vi "Create Section.vi"(8 "error in":errorcluster, 11 "Node In":refnum<k20>) -> (0 "error out":errorcluster, 2 "Section out":refnum<class "Section.lvclass">, 3 "Node out":refnum<k20>)   [LabVIEW 2024, in "Parser.lvlib" / "Section.lvclass"]
uses:
  Section.lvclass
  C:/Users/kperiyas/Downloads/Parser/Parser/Item/Item.lvclass
  Section.lvclass/Section.ctl
  Item/Item.lvclass/Item.ctl
  Item/Write Child Items.vi
  Item/Write Properties.vi
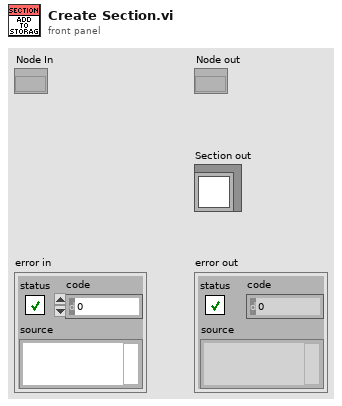
[diagram p1: front panel]
types:
  T1 = cluster{"Errors":cluster{"Key":string, "IsError":bool, "Code":u32, "Message":string}[], "Description":string}
  T2 = typedef "Parser.lvlib/Item.lvclass/Item Type.ctl" = enum16{"Channel", "Section"}
  T3 = cluster{"Name":string, "TypeGUID":string, "Identifier":string}
  T4 = cluster{"Key":string, "IsError":bool, "Code":u32, "Message":string}[]
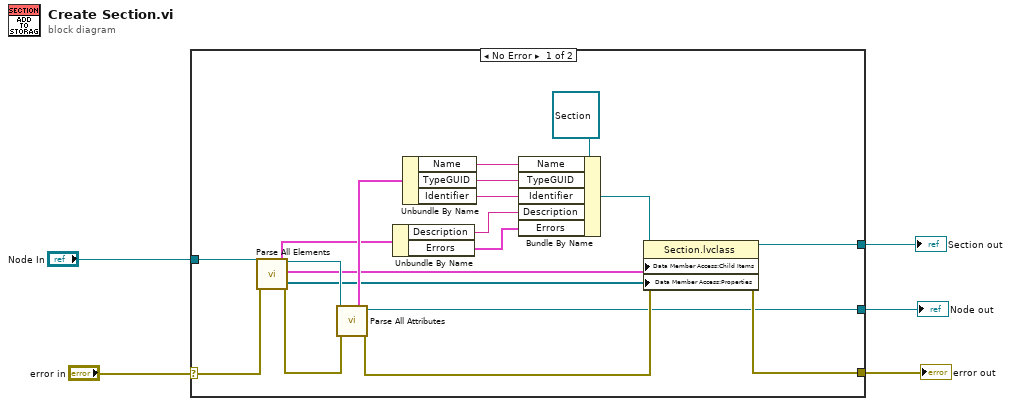
[diagram p0: block diagram]
diagram:
  n1 = case shown="No Error" "error in" {
    selector: "error in" -> [w24 w26]
    tunnel: [w21 w26] -> w4
    tunnel: "Node In" -> [w20 w25]
    tunnel: [w17 _] -> w2
    tunnel: [w6 w25] -> w1
    frame No Error {
      n2 = call "Parse All Elements.vi"("Node in"=w20, "error in"=w24) -> ("Node out"=w19:refnum<k20>, "Section Data"=w9:T1, "Child Items"=w8:cluster{"Item Type":T2, "Value":variant}[], "Properties out"=w7:refnum<class "Property.lvclass">[], "error out"=w23:errorcluster)  [unwired: 9 in]
      n3 = call "Parse All Attributes.vi"("error in"=w23, "Node In"=w19) -> ("error out"=w22:errorcluster, "Section Data"=w10:T3, "Node out"=w6:refnum<k20>)  [unwired: 7 in]
      n4 = Unbundle By Name(w9) -> ("Description"=w12:string, "Errors"=w11:T4)
      n5 = Unbundle By Name(w10) -> ("Name"=w18:string, "TypeGUID"=w16:string, "Identifier"=w15:string)
      n6 = Bundle By Name(cluster=refnum<class "Section.lvclass"> refnum ("Parser.lvlib:Section.lvclass"), "Name"=w18, "TypeGUID"=w16, "Identifier"=w15, "Description"=w12, "Errors"=w11) -> (w13:refnum<class "Section.lvclass">)
      n7 = property class="Section.lvclass"(reference=w13, error in=w22, "Data Member Access:Child Items"=w8, "Data Member Access:Properties"=w7) -> (reference out=w17:refnum<class "Section.lvclass">, error out=w21:errorcluster)
    }
    frame Error {
    }
  }
  "error out" <- w4
  "Section out" <- w2
  "Node out" <- w1
